vi "svx_Decimate Plots.vi"(7 "Cropped Info":cluster{"First Index":i32, "Length":i32}, 9 "Width":u32, 11 "Plots":cluster{"x0":dbl, "dx":dbl, "Y":dbl[]}[](array[cluster])) -> (3 "Plots out":cluster{"x0":dbl, "dx":dbl, "Y":dbl[]}[](array[cluster]))   [LabVIEW 2017, in "SVX Waterfall Graph.xctl"]
uses:
  <vilib>/addons/_XControls/Waterfall Graph/SVX Waterfall Graph.xctl
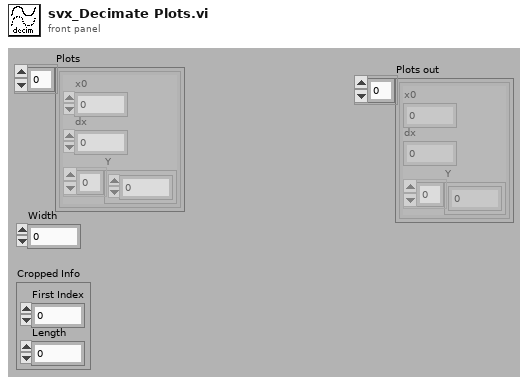
[diagram p1: front panel]
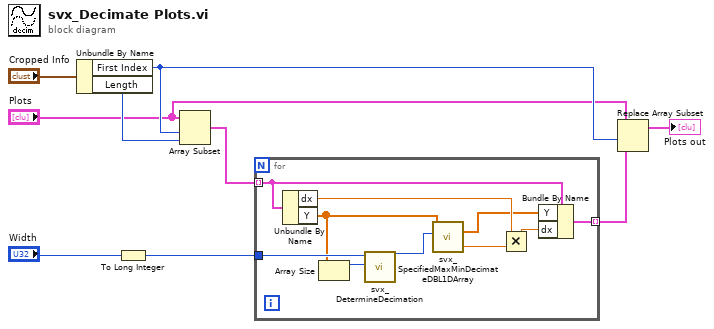
[diagram p0: block diagram]
diagram:
  n1 = Unbundle By Name("Cropped Info") -> ("First Index"=w6:i32, "Length"=w8:i32)
  n2 = To Long Integer(number="Width") -> (32bit integer=w1:i32)
  n3 = Array Subset(array="Plots", index=w6, length=w8) -> (w7:cluster{"x0":dbl, "dx":dbl, "Y":dbl[]}[])
  n4 = for {
    tunnel: w7 -> [w13] mode=indexing
    tunnel: w1 -> [w19]
    tunnel: [w10] -> w5 mode=indexing
    n5 = Unbundle By Name(w13) -> ("dx"=w15:dbl, "Y"=w17:dbl[])
    n6 = Array Size(array=w17) -> (size(s)=w18:i32)
    n7 = call <vilib>:"svx_DetermineDecimation.vi"("input buffer size"=w18, "display width"=w19) -> ("decimation\nfactor"=w16:i32)  [unwired: 6 in, 3 out]
    n8 = call <vilib>:"svx_SpecifiedMaxMinDecimateDBL1DArray.vi"("decimation factor"=w16, "DBL Array"=w17) -> ("actual decimation"=w14:dbl, "decimated array"=w12:dbl[])  [unwired: 7 in, 1 out]
    n9 = Multiply(x=w15, y=w14) -> (x*y=w11:dbl)
    n10 = Bundle By Name(cluster=w13, "Y"=w12, "dx"=w11) -> (w10:cluster{"x0":dbl, "dx":dbl, "Y":dbl[]})
  }
  n11 = Replace Array Subset(array="Plots", new element=w5, index=w6) -> (→"Plots out":cluster{"x0":dbl, "dx":dbl, "Y":dbl[]}[])
